vi "Read auth and create connection (SubVI).vi"(2 "error in (no error)":errorcluster, 3 "host name":string) -> (0 "error out":errorcluster, 1 "Connection out":refnum<class "Connection.lvclass">)   [LabVIEW 2016]
doc: "Read the authentification ~/.project8_authentications.json file and create a connection using the dripline informations in the sender_info global variable."
uses:
  <vilib>/Distrio/LabbitMQ/Connection/Connection.lvclass
panel:
  in  "Connection in":refnum<class "Connection.lvclass">
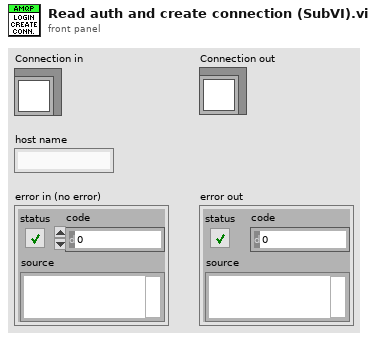
[diagram p1: front panel]
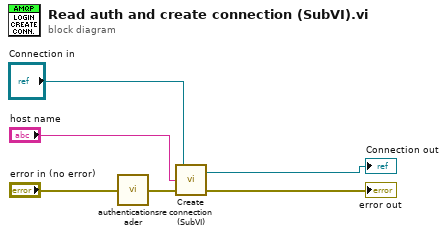
[diagram p0: block diagram]
diagram:
  n1 = call "authenticationsreader.vi"("error (in)"="error in (no error)") -> ("error (out)"=w1:errorcluster)
  n2 = call "Create connection (SubVI).vi"("error in (no error)"=w1, "host name"="host name", "Connection in"="Connection in") -> ("error out"=→"error out":errorcluster, "Connection out"=→"Connection out":refnum<class "Connection.lvclass">)
